vi "Save App Settings.vi"(8 "error in (no error)":errorcluster) -> (0 "error out":errorcluster)   [LabVIEW 2024, in "Data Base.lvlib"]
uses:
  Data Base.lvlib
  Support/General Type Defs/Global Data.vi
  <vilib>/Utility/config.llb/Write Key (Boolean).vi
  <vilib>/Utility/config.llb/Write Key (I32).vi
  <vilib>/Utility/config.llb/NI_LVConfig.lvlib
  Support/General Type Defs/General Type Definitions.lvlib
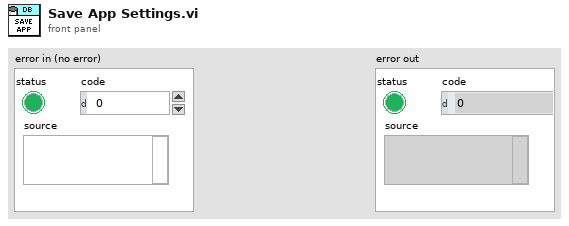
[diagram p1: front panel]
types:
  T1 = typedef "NI_LVConfig.lvlib/Config Data RefNum.ctl" = refnum<k1>
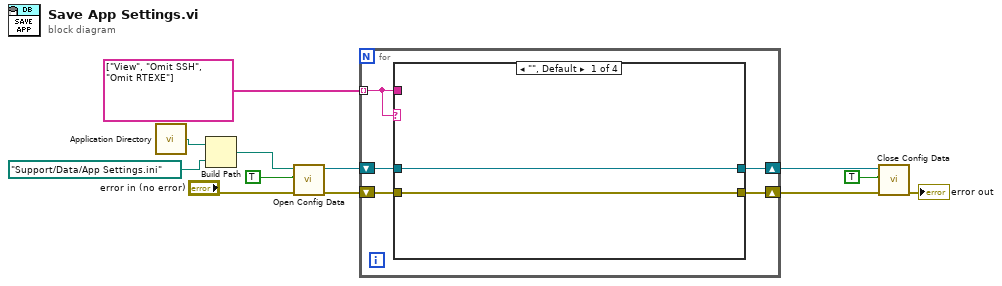
[diagram p0: block diagram]
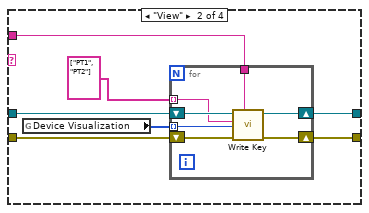
[diagram p2: hidden frame]
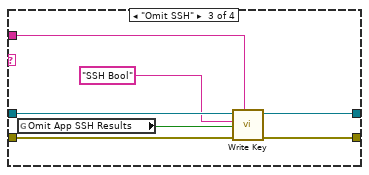
[diagram p3: hidden frame]
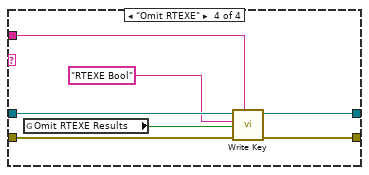
[diagram p4: hidden frame]
diagram:
  n1 = call <vilib>:"Application Directory.vi"() -> ("Application Directory"=w11:path)
  n2 = Build Path(base path=w11, name or relative path=path "Support/Data/App Settings.ini") -> (appended path=w6:path)
  n3 = call <vilib>:"Open Config Data.vi"("error in (no error)"="error in (no error)", "create file if necessary (T)"=TRUE, "configuration file path"=w6) -> ("error out"=w9:errorcluster, "refnum"=w10:T1)  [unwired: 6 in, 1 out]
  n4 = for {
    shift-right: [w15] -> w8
    shift-left: w10 -> [w17]
    shift-right: [w14] -> w7
    shift-left: w9 -> [w16]
    tunnel: string[] ["View", "Omit SSH", "Omit RTEXE"] -> [w13] mode=indexing
    n5 = case shown="\"\", Default" w13 {
      tunnel: w17 -> [w19 w26 w40 w47]
      tunnel: w16 -> [w18 w25 w39 w46]
      tunnel: [w19 w24 w38 w45] -> w15
      tunnel: [w18 w23 w37 w44] -> w14
      tunnel: w13 -> [_ w22 w36 w43]
      frame "", Default {
      }
      frame "View" {
        n6 = global read "Global Data.vi" "Device Visualization"() -> (w20:i32[])
        n7 = for {
          tunnel: w22 -> [w29]
          shift-right: [w31] -> w24
          shift-left: w26 -> [w33]
          shift-right: [w30] -> w23
          shift-left: w25 -> [w32]
          tunnel: string[] ["PT1", "PT2"] -> [w28] mode=indexing
          tunnel: w20 -> [w27] mode=indexing
          n8 = call-poly <vilib>:"Write Key.vi"("section"=w29, "error in (no error)"=w32, "value"=w27, "key"=w28, "refnum"=w33) -> ("error out"=w30:errorcluster, "refnum out"=w31:T1)  [unwired: 4 in, 1 out]
        }
      }
      frame "Omit SSH" {
        n9 = global read "Global Data.vi" "Omit App SSH Results"() -> (w34:bool)
        n10 = call-poly <vilib>:"Write Key.vi"("section"=w36, "error in (no error)"=w39, "value"=w34, "key"="SSH Bool", "refnum"=w40) -> ("error out"=w37:errorcluster, "refnum out"=w38:T1)  [unwired: 4 in, 1 out]
      }
      frame "Omit RTEXE" {
        n11 = global read "Global Data.vi" "Omit RTEXE Results"() -> (w41:bool)
        n12 = call-poly <vilib>:"Write Key.vi"("section"=w43, "error in (no error)"=w46, "value"=w41, "key"="RTEXE Bool", "refnum"=w47) -> ("error out"=w44:errorcluster, "refnum out"=w45:T1)  [unwired: 4 in, 1 out]
      }
    }
  }
  n13 = call <vilib>:"Close Config Data.vi"("error in (no error)"=w7, "write file if changed (T)"=TRUE, "refnum"=w8) -> ("error out"=→"error out":errorcluster)  [unwired: 7 in, 1 out]
